vi "WT-Ramp-Test.vi"() -> ()   [LabVIEW 2017]
uses:
  <vilib>/Platform/TimedLoop/XDataNode/timing_clust.ctl
  <vilib>/Platform/TimedLoop/XDataNode/nitl_modes.ctl
  <vilib>/Platform/TimedLoop/XDataNode/wakeup.ctl
  <vilib>/DAQmx/read.llb/DAQmx Read (Analog 1D DBL NChan 1Samp).vi
  <vilib>/DAQmx/miscellaneous.llb/DAQmx Fill In Error Info.vi
  <vilib>/express/express shared/transition.llb/Dynamic To Waveform Array.vi
  <vilib>/express/express signal manip/GetorSetDDTAttributes/Set DDT Attributes/SetT0.vi
  <vilib>/express/express shared/transition.llb/Waveform Array To Dynamic.vi
  <vilib>/platform/TimedLoop/XDataNode/XDataNode.xnode
  <vilib>/express/express signal manip/GetorSetDDTAttributes/Set DDT Attributes/Set DDT Properties.xnode
  <vilib>/measure/NI_MABase.lvlib
  <vilib>/Platform/TimedLoop/XDataNode/XDNodeRunTimeDep.lvlib
  <vilib>/Analysis/NI_AALPro.lvlib
panel:
  in  "upper limit":dbl=2.5 format="%#_13g"
  out "Waveform Chart":dbl(graph)
  in  "Stop Button":bool
  in  "ramps":i32=1
  in  "amplitude":dbl=1.0
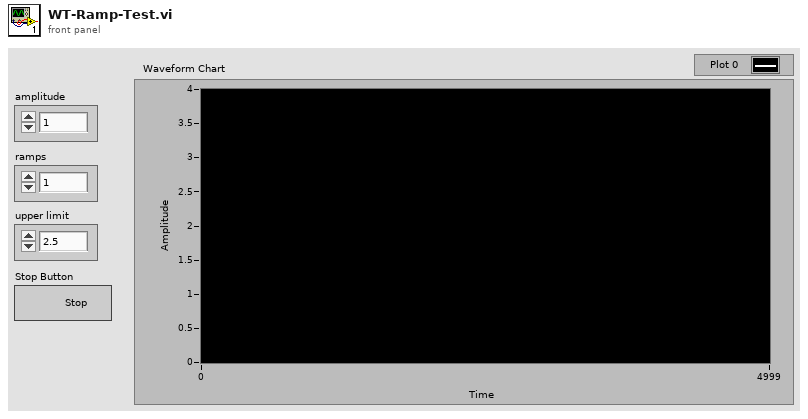
[diagram p1: front panel]
types:
  T1 = typedef "XDNodeRunTimeDep.lvlib/timing_clust.ctl" = cluster{"Expected End [f-1]":u64, "Actual End [f-1]":u64, "Finished Late? [f-1]":bool, "Expected End [i-1]":u64, "Actual End [i-1]":u64, "Finished Late? [i-1]":bool, "Expected Start [i]":u64, "Actual Start [i]":u64, "Expected Start [f]":u64, "Actual Start [f]":u64, "Source Name":string, "Structure Name":string, "Period":i64, "Deadline":i64, "Offset":i64, "Start":i64, "Priority":i32, "Timeout":i32, "Mode":T2, "Wakeup Reason":T3, "Error":errorcluster, "Source Type":string, "Secondary Source Type":string, "Global End Time":u64, "Global Start Time":u64, "Frame Duration":u64, "Iteration Duration":u64, "Assigned CPU":i32, "I/O Scan Engine Mode":u32}
  T2 = typedef "XDNodeRunTimeDep.lvlib/nitl_modes.ctl" = enum32{"No Change", "Process missed periods, maintain original phase", "Discard missed periods, maintain original phase", "Process missed periods, ignore original phase", "Discard missed periods, ignore original phase"}
  T3 = typedef "XDNodeRunTimeDep.lvlib/wakeup.ctl" = enum32{"Normal", "Aborted", "Asynchronous wakeup", "Timing source error", "Timed loop error", "Timeout"}
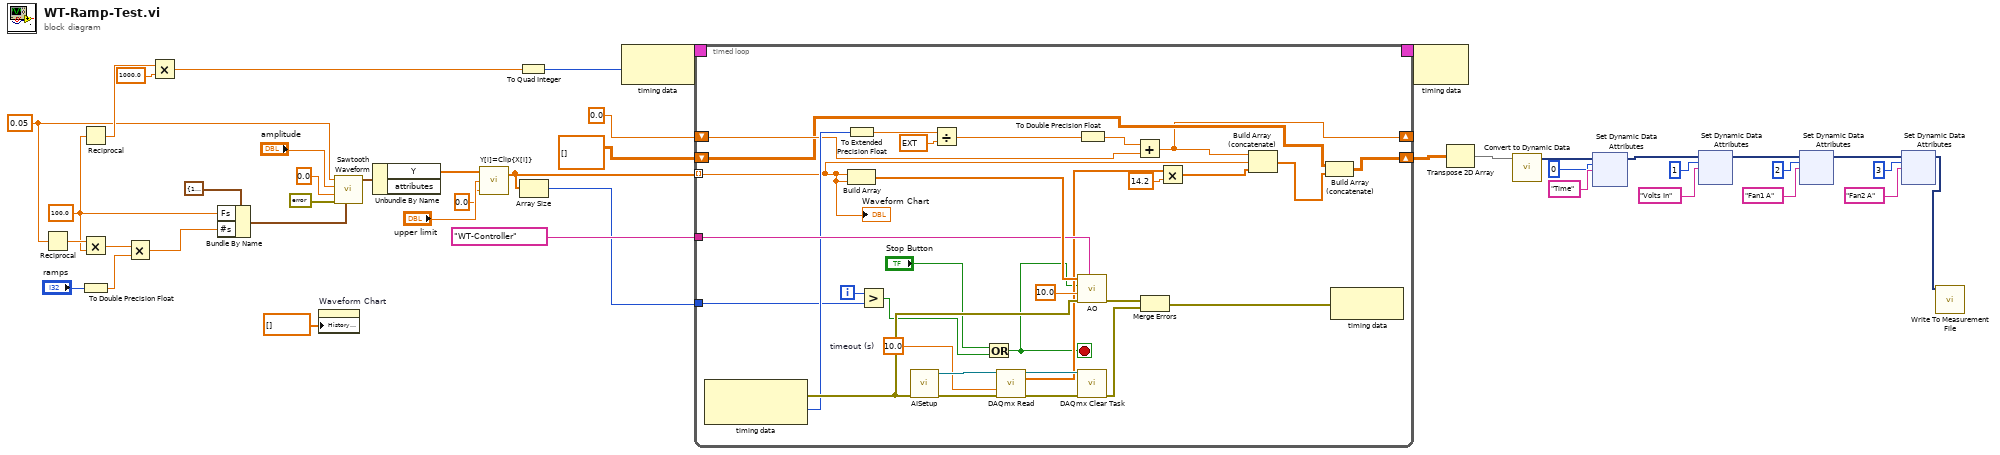
[diagram p0: block diagram]
diagram:
  w35 = 100.0 ("Fs")
  w37 = 0.05 ("frequency")
  n1 = Reciprocal(x=w37) -> (1/x=w36:dbl)
  n2 = Reciprocal(x=w35) -> (1/x=w40:dbl)
  n3 = Multiply(x=w36, y=w35) -> (x*y=w34:dbl)
  n4 = To Double Precision Float(number="ramps") -> (double precision float=w32:dbl)
  n5 = Multiply(x=w34, y=w32) -> (x*y=w31:dbl)
  n6 = Multiply(x=w40, y=1000.0) -> (x*y=w38:dbl)
  n7 = Bundle By Name(cluster=cluster{"Fs":dbl, "#s":dbl} {"Fs"=1000.0, "#s"=1000.0} ("sampling info"), "Fs"=w35, "#s"=w31) -> (w29:cluster{"Fs":dbl, "#s":dbl})
  n8 = property on="Waveform Chart" class="WFChart (strict)"("History Data"=dbl[] []) -> ()  [unwired: 2 in, 2 out]
  n9 = call <vilib>:"Sawtooth Waveform.vi"("sampling info"=w29, "error in (no error)"=errorcluster {"status"=FALSE, "code"=0, "source"=""}, "phase"=0.0, "amplitude"="amplitude", "frequency"=w37) -> ("signal out"=w28:waveform(dbl))  [unwired: 5 in, 1 out]
  n10 = Unbundle By Name(w28) -> ("Y"=w27:dbl[])  [unwired: 1 out]
  n11 = call <vilib>:"Y[i]=Clip{X[i]}.vi"("lower limit"=0.0, "upper limit"="upper limit", "Input Array"=w27) -> ("Clipped Array"=w4:dbl[])  [unwired: 1 out]
  n12 = To Quad Integer(1:w38) -> (0:w22:i64)
  n13 = Array Size(array=w4) -> (size(s)=w3:i32)
  n14 = node-c288(w22) -> (w24:T1)
  n15 = timed-loop {
    timing: w24 -> [_]
    timing-out: [_] -> w23
    tunnel: w4 -> [w53] mode=indexing
    tunnel: tag "WT-Controller" ("device name") -> [w73]
    shift-right: [w44] -> _
    shift-left: 0.0 -> [w59]
    shift-right: [w46] -> w5
    shift-left: dbl[][] [] -> [w45]
    tunnel: w3 -> [w51]
    i -> [w52]
    stop <- w48 stop-if-true
    w67 = 10.0  # timeout (s)
    n16 = node-c288() -> (w66:errorcluster, w62:i64)  [unwired: 1 in]
    n17 = To Extended Precision Float(1:w62) -> (0:w61:ext)
    n18 = Build Array(w53, w53) -> (w74:dbl[])
    n19 = Greater?(x=w52, y=w51) -> (0:w50:bool)
    n20 = call "AISetup.vi"("error in"=w66) -> ("error out"=w71:errorcluster, "task out"=w70:refnum<k21>)  [unwired: 9 in]
    n21 = Divide(x=w61, y=ext 1000.0) -> (x/y=w58:ext)
    n22 = Or(x="Stop Button", y=w50) -> (x .or. y?=w48:bool)
    n23 = call-poly <vilib>:"DAQmx Read.vi"("task/channels in"=w70, "timeout"=w67, "error in"=w71) -> ("task out"=w69:refnum<k21>, "data"=w55:dbl[], "error out"=w68:errorcluster)  [unwired: 10 in]
    n24 = call "AO.vi"("device name"=w73, "error in"=w66, "timeout (s)"=10.0, "stop (T)"=w48, "data"=w74) -> ("error out"=w65:errorcluster)  [unwired: 2 in, 1 out]
    n25 = call <vilib>:"DAQmx Clear Task.vi"("task in"=w69, "error in"=w68) -> ("error out"=w64:errorcluster)  [unwired: 13 in]
    n26 = To Double Precision Float(number=w58) -> (double precision float=w57:dbl)
    n27 = Add(x=w57, y=w59) -> (x+y=w44:dbl)
    n28 = Merge Errors(w65, w64) -> (w63:errorcluster)
    n29 = Multiply(x=w55, y=14.2) -> (x*y=w54:dbl[])
    n30 = Build Array (concatenate)(w44, w53, w54) -> (w47:dbl[])
    n31 = Build Array (concatenate)(w45, w47) -> (w46:dbl[][])
    n32 = node-c288(w63) -> ()  [unwired: 1 out]
    "Waveform Chart" <- w53
  }
  n33 = node-c288(w23) -> ()  [unwired: 1 out]
  n34 = Transpose 2D Array(2D array=w5) -> (transposed array=w7:dbl[][])
  n35 = call "Convert to Dynamic Data"("2D Array"=w7) -> ("Dynamic Data Type"=w6:dynamicdata)  [unwired: 3 in]
  n36 = xnode ("Set Dynamic Data Attributes")("Signals In"=w6, "Signal Index"=0, "Signal Name"="Time") -> ("Signals Out"=w10:dynamicdata)  [unwired: 1 in, 1 out]
  n37 = xnode ("Set Dynamic Data Attributes")("Signals In"=w10, "Signal Index"=1, "Signal Name"="Volts In") -> ("Signals Out"=w13:dynamicdata)  [unwired: 1 in, 1 out]
  n38 = xnode ("Set Dynamic Data Attributes")("Signals In"=w13, "Signal Index"=2, "Signal Name"="Fan1 A") -> ("Signals Out"=w14:dynamicdata)  [unwired: 1 in, 1 out]
  n39 = xnode ("Set Dynamic Data Attributes")("Signals In"=w14, "Signal Index"=3, "Signal Name"="Fan2 A") -> ("Signals Out"=w1:dynamicdata)  [unwired: 1 in, 1 out]
  n40 = call "Write To Measurement File"("Signals"=w1) -> ()  [unwired: 16 in, 3 out]
